vi "DTV&EnQueue.vi"(0 "ModuleAdmin In":refnum<class "ModuleAdmin.lvclass">, 2 "Enqueue Type (Enqueue)":T2=enum."Enqueue", 5 "Message":string, 7 "Message Data":variant, 9 "Class":refnum<class "AnalysisPluginsBase.lvclass">, 11 "Error In":errorcluster, 13 "QueueArrayEntry(QMH)":T1) -> (4 "ModuleAdmin Out":refnum<class "ModuleAdmin.lvclass">, 6 "MessageQueue Out":refnum<queue>, 8 "Varia\nntData":variant, 15 "Error Out":errorcluster)   [LabVIEW 2018, in "AnalysisModule.lvlib"]
uses:
  AnalysisModule.lvlib
  <userlib>/NIST/ModuleAdminLib/ModuleAdmin/ModuleAdmin.lvclass
  <userlib>/NIST/ModuleAdminLib/ModuleAdmin/TypeDefinitions/QueueType.ctl
  AnalysisPlugins/AnalysisPluginBaseClass/AnalysisPluginsBase.lvclass
  <userlib>/NIST/ModuleAdminLib/ModuleAdmin/TypeDefinitions/QueueEntry.ctl
  clAnalysisMsg.ctl
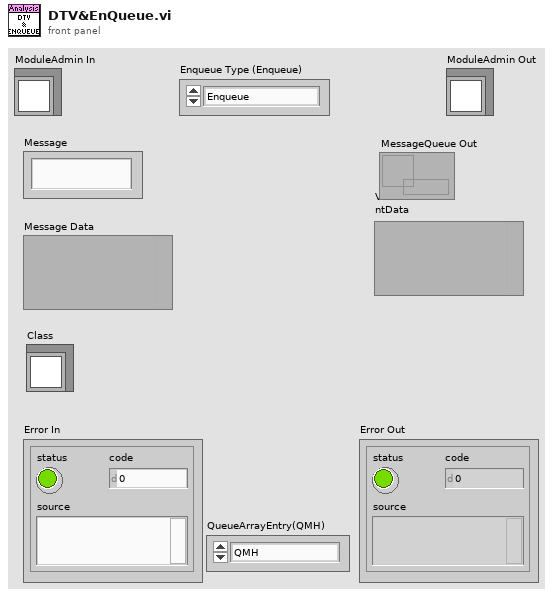
[diagram p1: front panel]
types:
  T1 = typedef "ModuleAdmin.lvlib/ModuleAdmin.lvclass/QueueEntry.ctl" = enum16{"QMH", "Class Data", "Data Loop", "Queue 4", "Queue 5", "Queue 6", "Queue 7", "Queue 8", "Queue 9", "Queue 10"}
  T2 = typedef "ModuleAdmin.lvlib/ModuleAdmin.lvclass/QueueType.ctl" = enum16{"EnqueueAtFront", "Enqueue", "Lossy Enqueue"}
  T3 = typedef "AnalysisModule.lvlib/clAnalysisMsg.ctl" = cluster{"Class":refnum<class "AnalysisPluginsBase.lvclass">, "Message":string, "Message Data":variant}
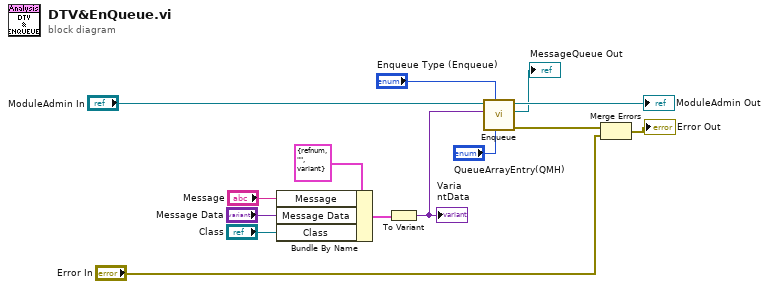
[diagram p0: block diagram]
diagram:
  n1 = Bundle By Name(cluster=T3 {"Class"=refnum, "Message"="", "Message Data"=variant} ("clAnalysisMsg"), "Message"="Message", "Message Data"="Message Data", "Class"="Class") -> (w7:T3)
  n2 = To Variant(anything=w7) -> (Variant=w5:variant)
  "Varia\nntData" <- w5
  n3 = call <userlib>:"Enqueue.vi"("QueueArrayEntry(QMH)"="QueueArrayEntry(QMH)", "Enqueue Type (Enqueue)"="Enqueue Type (Enqueue)", "Queue Element"=w5, "ModuleAdmin In"="ModuleAdmin In") -> ("error out"=w12:errorcluster, "MessageQueue Out"=→"MessageQueue Out":refnum<queue>, "ModuleAdmin Out"=→"ModuleAdmin Out":refnum<class "ModuleAdmin.lvclass">)  [unwired: 5 in]
  n4 = Merge Errors(w12, "Error In") -> (→"Error Out":errorcluster)
